vi "lzs1.vi"() -> ()   [LabVIEW 2014]
panel:
  out "添加的路径":path
  out "standard error":string caption="标准错误"
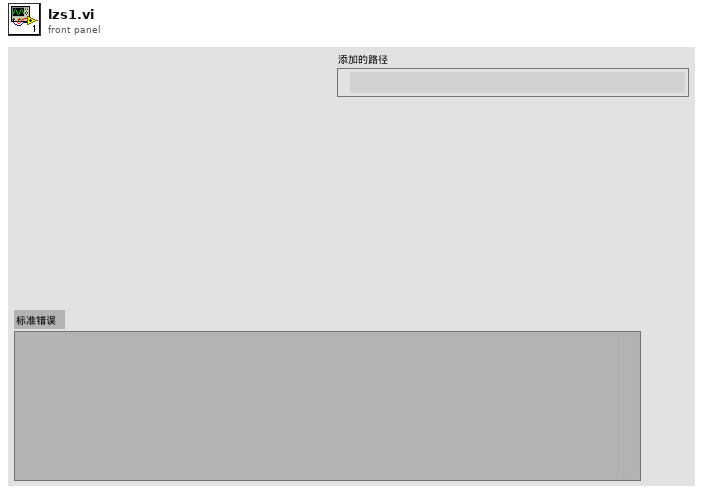
[diagram p1: front panel]
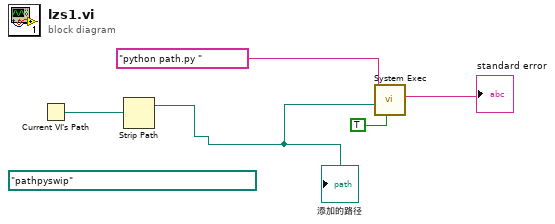
[diagram p0: block diagram]
diagram:
  (unwired) path "pathpyswip"
  n1 = Current VI's Path() -> (path=w2:path)
  n2 = Strip Path(path=w2) -> (stripped path=w1:path)  [unwired: 1 out]
  "添加的路径" <- w1
  n3 = call <vilib>:"System Exec.vi"("run minimized? (F)"=TRUE, "working directory"=w1, "command line"="python path.py ") -> ("standard error"=→"standard error":string)  [unwired: 5 in, 3 out]
